vi "Convert Filter to Display String.vi"(11 "Filter Info":T1={"Filter Column"=enum."Description", "Filter Type"=enum."Contains", "Filter Value"="", "New Data?"=FALSE, "Case Sensitive?"=FALSE, "Enabled?"=FALSE}) -> (3 "String":string)   [LabVIEW 2020, in "VI Properties Editor.lvlib"]
doc: "Converts <B>Filter Info<B> to a string to be displayed."
uses:
  VI Properties Editor.lvlib
  CTLs/Filter Info.ctl
  CTLs/Filter Column.ctl
  CTLs/Filter Type.ctl
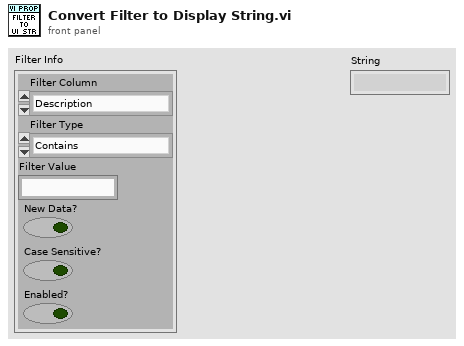
[diagram p1: front panel]
types:
  T1 = typedef "VI Properties Editor.lvlib/Filter Info.ctl" = cluster{"Filter Column":T2, "Filter Type":T3, "Filter Value":string, "New Data?":bool, "Case Sensitive?":bool, "Enabled?":bool}
  T2 = typedef "VI Properties Editor.lvlib/Filter Column.ctl" = enum16{"Name", "Path", "Type", "Window Title", "Description", "Help Path", "Help Tag", "Custom Title?", "Reentrancy", "Inlined?", "Help URL", "Help Type", "Allow Debugging?", "Auto Error Handling?", "Run When Opened?", "Suspend When Called?", "Priority", "Preferred Exec Sytem", "Control Label", "Control Caption", "Control Description", "Control Tip Strip"}
  T3 = typedef "VI Properties Editor.lvlib/Filter Type.ctl" = enum16{"Contains", "Equals", "Starts with", "Ends with", "Is empty", "Does not contain", "Does not equal", "Is not empty"}
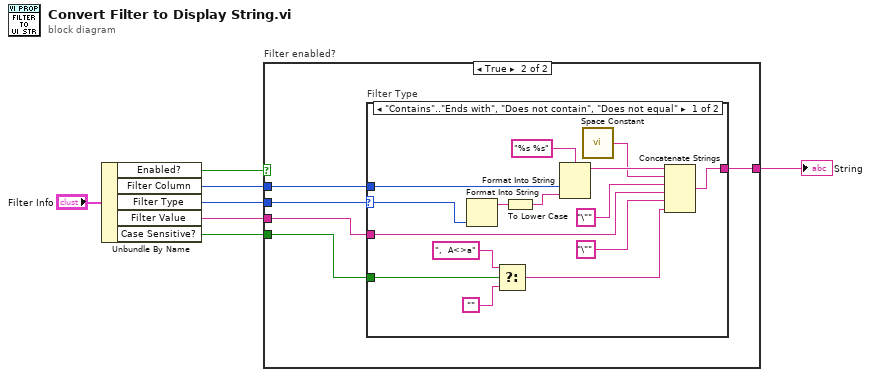
[diagram p0: block diagram]
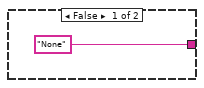
[diagram p2: hidden frame]
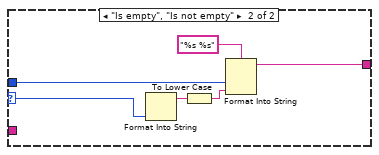
[diagram p3: hidden frame]
diagram:
  n1 = Unbundle By Name("Filter Info") -> ("Enabled?"=w2:bool, "Filter Column"=w4:T2, "Filter Type"=w6:T3, "Filter Value"=w5:string, "Case Sensitive?"=w1:bool)
  n2 = case "Filter enabled?" shown="True" w2 {
    tunnel: w6 -> [_ w13]
    tunnel: w5 -> [_ w12]
    tunnel: w4 -> [_ w11]
    tunnel: ["None" w10] -> w3
    tunnel: w1 -> [_ w9]
    frame False {
    }
    frame True {
      n3 = case "Filter Type" shown="\"Contains\"..\"Ends with\", \"Does not contain\", \"Does not equal\"" w13 {
        selector: w13 -> [w25 w31]
        tunnel: w12 -> [w21 _]
        tunnel: w11 -> [w27 w33]
        tunnel: [w18 w32] -> w10
        tunnel: w9 -> [w17 _]
        frame "Contains".."Ends with", "Does not contain", "Does not equal" {
          n4 = Format Into String(w25) -> (resulting string=w26:string)  [unwired: 3 in, 1 out]
          n5 = Select(t=",  A<>a", s=w17, f="") -> (s? t:f=w15:string)
          n6 = To Lower Case(string=w26) -> (all lower case string=w24:string)
          n7 = Format Into String(format string="%s %s", w27, w24) -> (resulting string=w23:string)  [unwired: 2 in, 1 out]
          n8 = call <vilib>:"Space Constant.vi"() -> ("String"=w22:string)
          n9 = Concatenate Strings(w23, w22, "\"", w21, "\"", w15) -> (w18:string)
        }
        frame "Is empty", "Is not empty" {
          n10 = Format Into String(w31) -> (resulting string=w30:string)  [unwired: 3 in, 1 out]
          n11 = To Lower Case(string=w30) -> (all lower case string=w29:string)
          n12 = Format Into String(format string="%s %s", w33, w29) -> (resulting string=w32:string)  [unwired: 2 in, 1 out]
        }
      }
    }
  }
  "String" <- w3
